vi "Render Recusive Partial with Single Recursion.vi"(8 "Error In":errorcluster) -> (0 "Error Out":errorcluster)   [LabVIEW 2018, in "Tests.lvlib" / "Render.lvlib"]
uses:
  Render.lvlib
  <vilib>/addons/_JKI Toolkits/Caraya/classes/Test/Test.lvclass
  <vilib>/addons/_JKI Toolkits/Caraya/classes/Assert/Assert.lvclass
  src/Toolkit/Low-Level/Loaders/String/String.lvclass
  src/Toolkit/Data/Pair/Pair.lvclass
  src/Toolkit/Data/Pair/Support/From String.vi
  src/Toolkit/Data/Array/Array.lvclass
  src/Toolkit/Data/Map/Map.lvclass
  src/Toolkit/Data/Pair/Support/From Datum.vi
  src/Toolkit/Data/Map/Support/From Pair Array.vi
  D:/Users/cfield/Code/Field R&D Services/Labstache/src/Toolkit/Data/Datum/Datum.lvclass
  src/Toolkit/Data/Array/Support/From Strings.vi
  src/Toolkit/Data/Array/Support/From Data.vi
  src/Toolkit/Low-Level/Support/Lex String.vi
  src/Toolkit/Low-Level/Renderer/Abstract/Render to String.vi
  src/Toolkit/Low-Level/Compiler/Compiler.lvclass
  D:/Users/cfield/Code/Field R&D Services/Labstache/src/Toolkit/Low-Level/Loaders/Loader/Loader.lvclass
  src/Toolkit/Low-Level/Nodes/Root/Root.lvclass
  D:/Users/cfield/Code/Field R&D Services/Labstache/src/Toolkit/Low-Level/Nodes/NonTerminal/NonTerminal.lvclass
  D:/Users/cfield/Code/Field R&D Services/Labstache/src/Toolkit/Low-Level/Nodes/Node/Node.lvclass
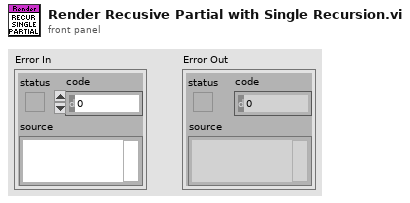
[diagram p1: front panel]
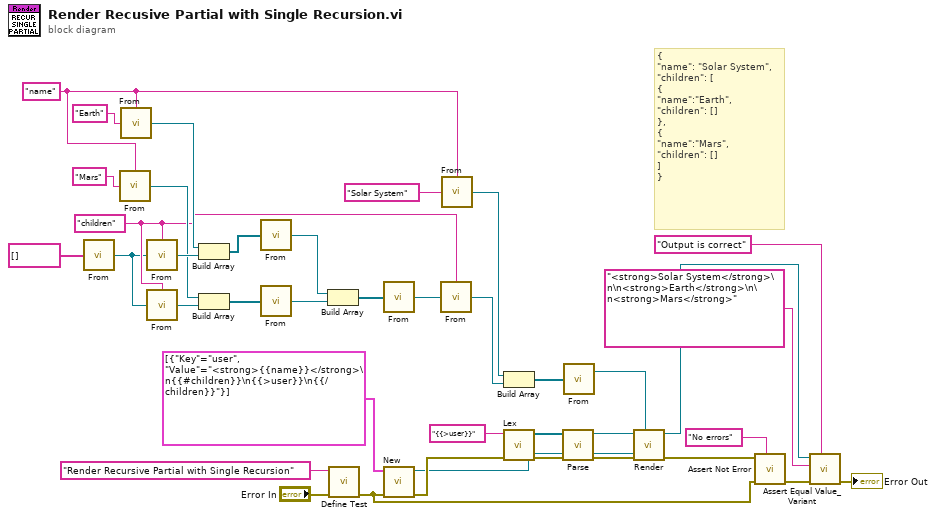
[diagram p0: block diagram]
diagram:
  w3 = "children" ("Key")
  w4 = "name" ("Key")
  # "{\n\"name\": \"Solar System\",\n\"children\": [\n{\n\"name\":\"Earth\",\n\"children\": []\n},\n{\n\"name\":\"Mars\",\n\"children\": []\n]\n}"
  n1 = call-poly "From.vi"("Strings"=string[] []) -> ("Array"=w1:refnum<class "Array.lvclass">)  [unwired: 1 in]
  n2 = call-poly "From.vi"("Value"="Mars", "Key"=w4) -> ("Pair"=w8:refnum<class "Pair.lvclass">)
  n3 = call-poly "From.vi"("Value"="Earth", "Key"=w4) -> ("Pair"=w13:refnum<class "Pair.lvclass">)
  n4 = call-poly "From.vi"("Value"=w1, "Key"=w3) -> ("Pair"=w12:refnum<class "Pair.lvclass">)
  n5 = call-poly "From.vi"("Value"=w1, "Key"=w3) -> ("Pair"=w7:refnum<class "Pair.lvclass">)
  n6 = Build Array(w13, w12) -> (w11:refnum<class "Pair.lvclass">[])
  n7 = Build Array(w8, w7) -> (w6:refnum<class "Pair.lvclass">[])
  n8 = call-poly "From.vi"("Pairs"=w11) -> ("Map"=w10:refnum<class "Map.lvclass">)  [unwired: 1 in]
  n9 = call-poly "From.vi"("Pairs"=w6) -> ("Map"=w2:refnum<class "Map.lvclass">)  [unwired: 1 in]
  n10 = Build Array(w10, w2) -> (w19:refnum<class "Map.lvclass">[])
  n11 = call <vilib>:"Define Test.vi"("error in (no error)"="Error In", "Label (VI Title)"="Render Recursive Partial with Single Recursion") -> ("error out"=w25:errorcluster)  [unwired: 9 in]
  n12 = call-poly "From.vi"("Data"=w19) -> ("Array"=w18:refnum<class "Array.lvclass">)  [unwired: 1 in]
  n13 = call "New.vi"("Error In"=w25, "Key-Value Pairs"=cluster{"Key":string, "Value":string}[] [{"Key"="user", "Value"="<strong>{{name}}</strong>\n{{#children}}\n{{>user}}\n{{/children}}"}]) -> ("Error Out"=w27:errorcluster, "String"=w22:refnum<class "String.lvclass">)  [unwired: 8 in]
  n14 = call-poly "From.vi"("Value"=w18, "Key"=w3) -> ("Pair"=w16:refnum<class "Pair.lvclass">)
  n15 = call-poly "From.vi"("Value"="Solar System", "Key"=w4) -> ("Pair"=w17:refnum<class "Pair.lvclass">)
  n16 = Build Array(w17, w16) -> (w15:refnum<class "Pair.lvclass">[])
  n17 = call-poly "Lex.vi"("Error In"=w27, "Input"="{{>user}}" ("format string")) -> ("Error Out"=w29:errorcluster, "Tokens"=w30:refnum<class "Token.lvclass">[])  [unwired: 8 in]
  n18 = call "Parse.vi"("Error In"=w29, "Tokens"=w30) -> ("Error Out"=w31:errorcluster, "Abstract Syntax Tree"=w28:refnum<class "Root.lvclass">)  [unwired: 8 in]
  n19 = call-poly "From.vi"("Pairs"=w15) -> ("Map"=w14:refnum<class "Map.lvclass">)  [unwired: 1 in]
  n20 = call-poly "Render.vi"(6:w22, 7:w14, "Error In"=w31, "Context In"=w28) -> ("Error Out"=w33:errorcluster, "Context Out"=w32:refnum<class "Compiler.lvclass">)  [unwired: 5 in, 1 out]
  n21 = call <vilib>:"Assert Not Error.vi"("Label"="No errors", "error in (no error)"=w25, "Not Error?"=w33) -> ("error out"=w36:errorcluster)  [unwired: 8 in]
  n22 = call <vilib>:"Assert Equal Value_Variant.vi"("Label"="Output is correct", "error in (no error)"=w36, "Y"="<strong>Solar System</strong>\n\n<strong>Earth</strong>\n\n<strong>Mars</strong>", "X"=w32) -> ("error out"=→"Error Out":errorcluster)  [unwired: 7 in]
